vi "Partial Derivative Prep.vi"(0 "formula":string, 1 "End":dbl[](array[numeric])=[1.0, 1.0] format="%.2f", 5 "Variables":string[](array[string])=["x1", "x2"], 7 "Start":dbl[](array[numeric])=[0.0, 0.0] format="%.2f", 9 "derivative":u16(ring) items=["first variable", "second variable"]) -> (4 "Variables":string[](array[string]), 6 "formula":string, 8 "End":dbl[](array[numeric]) format="%.2f", 10 "?":u32, 11 "derivative":u16, 12 "Start":dbl[](array[numeric]) format="%.2f", 13 "specific error 2":bool, 14 "error (general)":bool, 15 "specific error 1":bool)   [LabVIEW 2017, in "NI_Gmath.lvlib"]
uses:
  NI_Gmath.lvlib
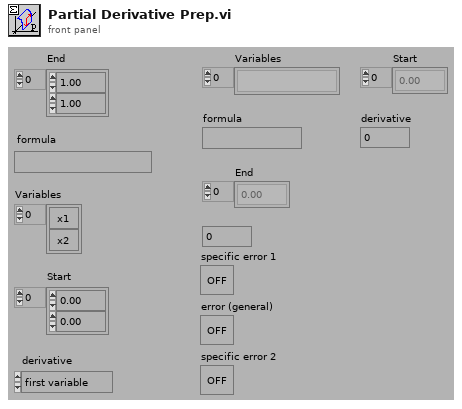
[diagram p1: front panel]
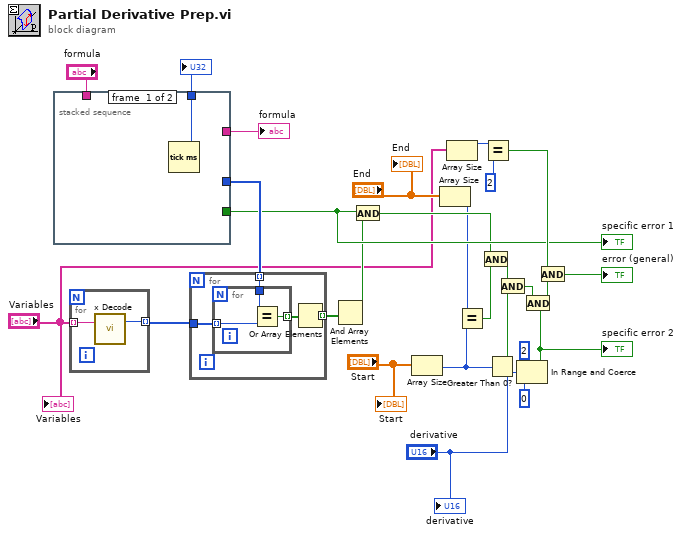
[diagram p0: block diagram]
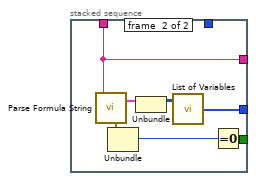
[diagram p2: hidden frame]
diagram:
  n1 = stacked-sequence {
    tunnel: [_ w35] -> w19
    tunnel: [w28 _] -> w4
    tunnel: [_ w34] -> w21
    tunnel: [_ w33] -> w3
    tunnel: "formula" -> [_ w33]
    frame #0 {
      n2 = Tick Count (ms)() -> (millisecond timer value=w28:u32)
    }
    frame #1 {
      n3 = call "Parse Formula String.vi"("formula"=w33) -> ("error out"=w32:errorcluster, "Parsed Formula"=w30:cluster{"Table":i32[][], "Y Values":dbl[]})  [unwired: 1 in]
      n4 = Unbundle(w32) -> ("code"=w31:i32)  [unwired: 2 out]
      n5 = Unbundle(w30) -> ("Table"=w29:i32[][])  [unwired: 1 out]
      n6 = call "List of Variables.vi"("Table"=w29) -> ("List of variables"=w34:i32[])
      n7 = Equal To 0?(x=w31) -> (x = 0?=w35:bool)
    }
  }
  "specific error 1" <- w19
  "?" <- w4
  "formula" <- w3
  n8 = for {
    tunnel: "Variables" -> [w37] mode=indexing
    tunnel: [w36] -> w20 mode=indexing
    n9 = call "x Decode.vi"("x string"=w37) -> ("number"=w36:i32)  [unwired: 1 in, 1 out]
  }
  n10 = for {
    tunnel: [w40] -> w22 mode=indexing
    tunnel: w21 -> [w39] mode=indexing
    tunnel: w20 -> [w38]
    n11 = for {
      tunnel: [w44] -> w41 mode=indexing
      tunnel: w39 -> [w43]
      tunnel: w38 -> [w42] mode=indexing
      n12 = Equal?(x=w43, y=w42) -> (x = y?=w44:bool)
    }
    n13 = Or Array Elements(Boolean array=w41) -> (logical OR=w40:bool)
  }
  n14 = And Array Elements(Boolean array=w22) -> (logical AND=w2:bool)
  n15 = And(x=w19, y=w2) -> (x .and. y?=w13:bool)
  n16 = Array Size(array="Start") -> (size(s)=w8:i32)
  n17 = Array Size(array="End") -> (size(s)=w6:i32)
  n18 = Array Size(array="Variables") -> (size(s)=w23:i32)
  n19 = Equal?(x=w6, y=w8) -> (x = y?=w7:bool)
  n20 = And(x=w13, y=w7) -> (x .and. y?=w10:bool)
  n21 = Equal?(x=w23, y=2) -> (x = y?=w25:bool)
  n22 = Greater Than 0?(x=w8) -> (x > 0?=w9:bool)
  n23 = And(x=w10, y=w9) -> (x .and. y?=w17:bool)
  n24 = In Range and Coerce(upper limit=2, x="derivative", lower limit=0) -> (In Range?=w18:bool)  [unwired: 1 out]
  "specific error 2" <- w18
  n25 = And(x=w17, y=w18) -> (x .and. y?=w26:bool)
  n26 = And(x=w25, y=w26) -> (x .and. y?=→"error (general)":bool)
  "Variables" <- "Variables"
  "derivative" <- "derivative"
  "Start" <- "Start"
  "End" <- "End"
